vi "写入路径.vi"(8 "error in (no error)":errorcluster caption="错误输入（无错误）", 10 "路径":path, 11 "RunningLog输入":refnum<class "RunningLog.lvclass">) -> (0 "error out":errorcluster caption="错误输出", 3 "RunningLog输出":refnum<class "RunningLog.lvclass">)   [LabVIEW 2018, in "RunningLog.lvclass"]
uses:
  RunningLog.lvclass
  RunningLog.lvclass/RunningLog.ctl
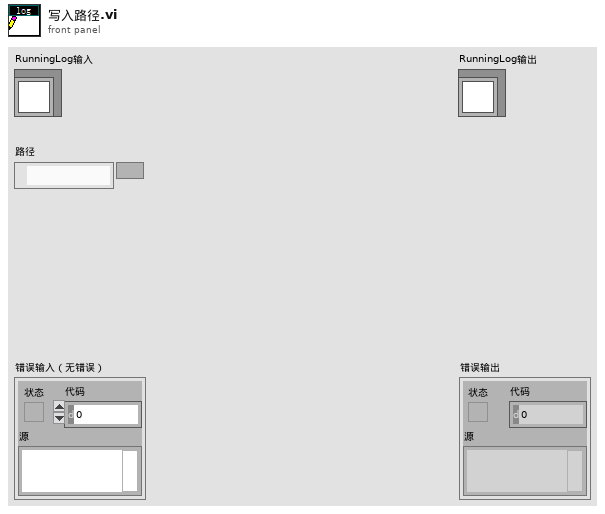
[diagram p1: front panel]
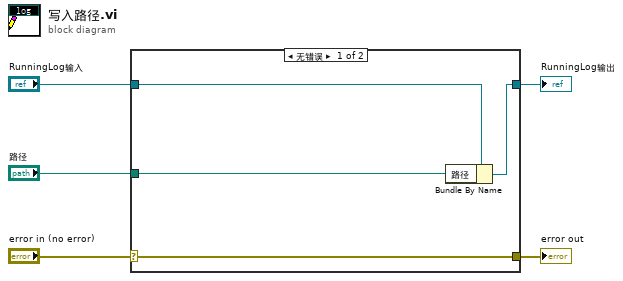
[diagram p0: block diagram]
diagram:
  n1 = case shown="无错误" "error in (no error)" {
    selector: "error in (no error)" -> [w9 w10]
    tunnel: [w9 w10] -> w4
    tunnel: [w7 w11] -> w2
    tunnel: "RunningLog输入" -> [w8 w11]
    tunnel: "路径" -> [w6 _]
    frame No Error {
      n2 = Bundle By Name(cluster=w8, "路径"=w6) -> (w7:refnum<class "RunningLog.lvclass">)
    }
    frame Error {
    }
  }
  "error out" <- w4
  "RunningLog输出" <- w2
